vi "Top_and_Tail_ph.vi"(2 "Array in":dbl[](array[numeric]), 3 "Threshold":dbl) -> (0 "Length":i32, 1 "Start Index":i32)   [LabVIEW 2010]
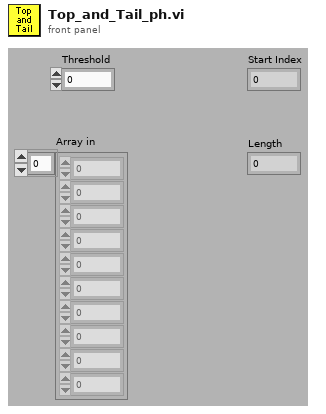
[diagram p1: front panel]
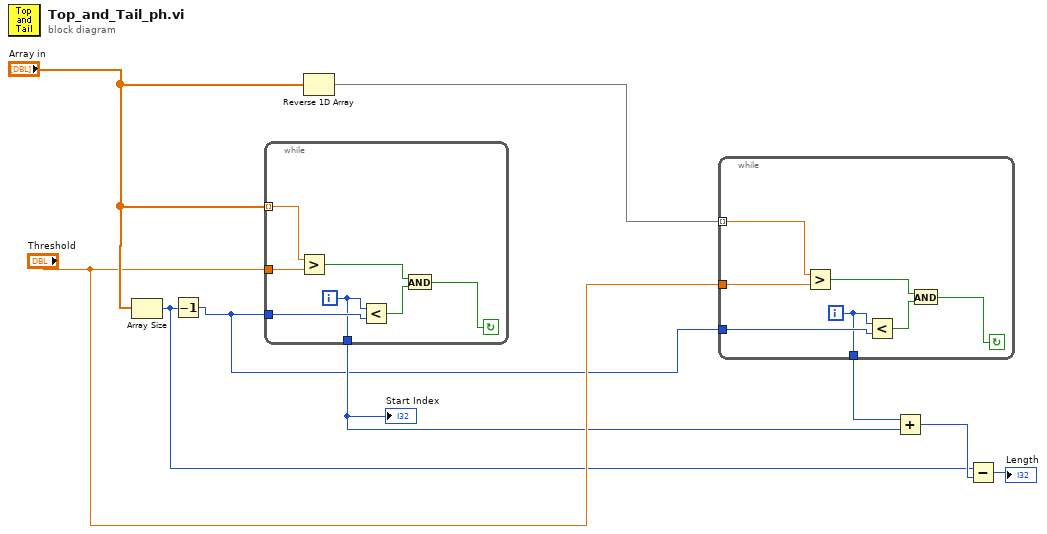
[diagram p0: block diagram]
diagram:
  n1 = Array Size(array="Array in") -> (size(s)=w3:i32)
  n2 = Decrement(x=w3) -> (x-1=w2:i32)
  n3 = while {
    tunnel: "Array in" -> [w16] mode=indexing
    tunnel: "Threshold" -> [w15]
    tunnel: w2 -> [w14]
    tunnel: [w10] -> w5
    i -> [w10]
    stop <- w11 continue-if-true
    n4 = Greater?(x=w16, y=w15) -> (0:w13:bool)
    n5 = Less?(x=w10, y=w14) -> (x < y?=w12:bool)
    n6 = And(x=w13, y=w12) -> (x .and. y?=w11:bool)
  }
  "Start Index" <- w5
  n7 = Reverse 1D Array(array="Array in") -> (reversed array=w7:dbl[])
  n8 = while {
    tunnel: w7 -> [w23] mode=indexing
    tunnel: "Threshold" -> [w22]
    tunnel: w2 -> [w21]
    tunnel: [w17] -> w6
    i -> [w17]
    stop <- w18 continue-if-true
    n9 = Greater?(x=w23, y=w22) -> (0:w20:bool)
    n10 = Less?(x=w17, y=w21) -> (x < y?=w19:bool)
    n11 = And(x=w20, y=w19) -> (x .and. y?=w18:bool)
  }
  n12 = Add(x=w6, y=w5) -> (x+y=w4:i32)
  n13 = Subtract(x=w3, y=w4) -> (x-y=→"Length":i32)
